vi "2022_day8_sub_evaluate_tree_visibility.vi"(1 "Tree Sizes Map":i32[][](array[numeric])) -> (0 "Visible Trees Map":bool[][](array[boolean]))   [LabVIEW 2021]
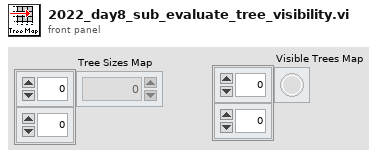
[diagram p1: front panel]
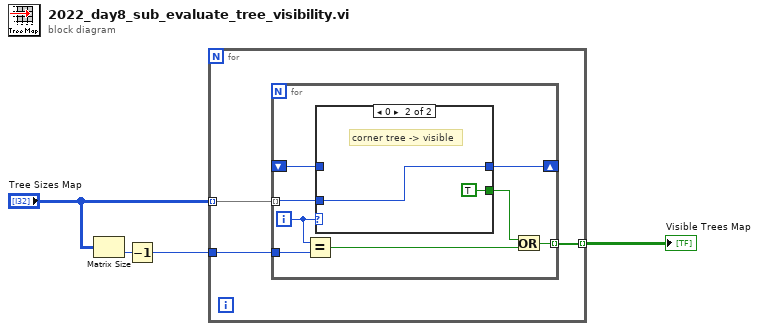
[diagram p0: block diagram]
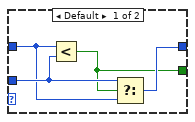
[diagram p2: hidden frame]
diagram:
  n1 = Matrix Size(0:"Tree Sizes Map") -> (2:w2:i32)  [unwired: 1 out]
  n2 = Decrement(x=w2) -> (x-1=w4:i32)
  n3 = for {
    tunnel: "Tree Sizes Map" -> [w7] mode=indexing
    tunnel: [w6] -> w3 mode=indexing
    tunnel: w4 -> [w5]
    n4 = for {
      tunnel: w7 -> [w13] mode=indexing
      tunnel: [w15] -> w6 mode=indexing
      shift-right: [w12] -> _
      shift-left: _ -> [w11]
      tunnel: w5 -> [w9]
      i -> [w14]
      n5 = Equal?(x=w14, y=w9) -> (x = y?=w8:bool)
      n6 = case shown="0" w14 {
        tunnel: w13 -> [w19 w21]
        tunnel: [w18 w21] -> w12
        tunnel: w11 -> [w17 _]
        tunnel: [w16 TRUE] -> w10
        frame Default {
          n7 = Less?(x=w17, y=w19) -> (x < y?=w16:bool)
          n8 = Select(t=w19, s=w16, f=w17) -> (s? t:f=w18:i32)
        }
        frame 0 {
          # "corner tree -> visible"
        }
      }
      n9 = Or(x=w10, y=w8) -> (x .or. y?=w15:bool)
    }
  }
  "Visible Trees Map" <- w3
